vi "Combine Litho Data.vi"(8 "error in (no error)":errorcluster, 11 "Tool Object in":refnum<class "Tool Object.lvclass">) -> (0 "error out":errorcluster, 2 "Output":T1(array[cluster]), 3 "Tool Object out":refnum<class "Tool Object.lvclass">)   [LabVIEW 2019, in "Tool Object.lvclass"]
uses:
  Tool Object.lvclass
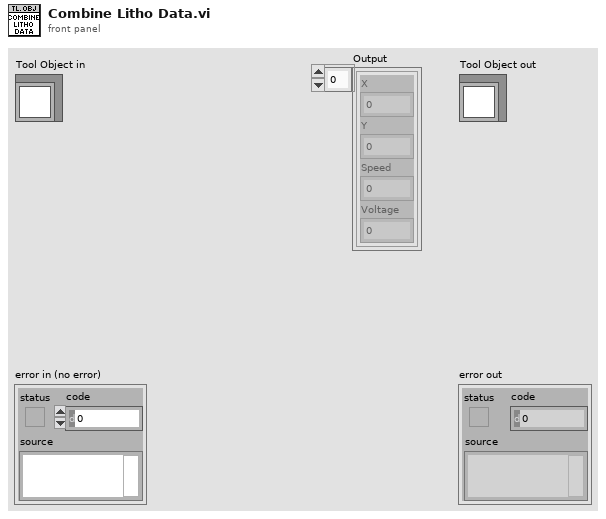
[diagram p1: front panel]
types:
  T1 = cluster{"X":dbl, "Y":dbl, "Speed":dbl, "Voltage":dbl}[]
  T2 = typedef "PathCommands.lvclass/Point.ctl" = cluster{"X":dbl, "Y":dbl}
  T3 = cluster{"X":dbl, "Y":dbl, "Speed":dbl, "Voltage":dbl}
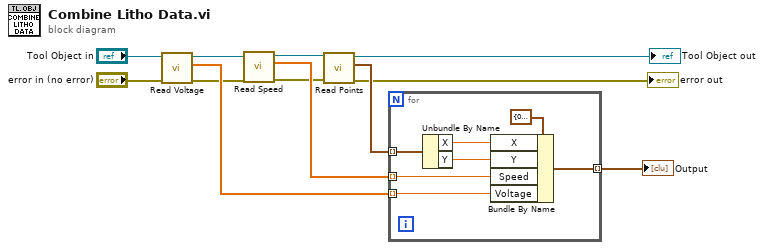
[diagram p0: block diagram]
diagram:
  n1 = call-dynamic "Read Voltage.vi"("error in (no error)"="error in (no error)", "Tool Object in"="Tool Object in") -> ("error out"=w4:errorcluster, "Voltage"=w6:dbl[], "Tool Object out"=w8:refnum<class "Tool Object.lvclass">)  [unwired: 7 in]
  n2 = call-dynamic "Read Speed.vi"("error in (no error)"=w4, "Tool Object in"=w8) -> ("error out"=w3:errorcluster, "Speed"=w5:dbl[], "Tool Object out"=w9:refnum<class "Tool Object.lvclass">)  [unwired: 7 in]
  n3 = call-dynamic "Read Points.vi"("error in (no error)"=w3, "Tool Object in"=w9) -> ("error out"=→"error out":errorcluster, "Points"=w12:T2[], "Tool Object out"=→"Tool Object out":refnum<class "Tool Object.lvclass">)  [unwired: 7 in]
  n4 = for {
    tunnel: w5 -> [w15] mode=indexing
    tunnel: w12 -> [w19] mode=indexing
    tunnel: w6 -> [w14] mode=indexing
    tunnel: [w13] -> w11 mode=indexing
    n5 = Unbundle By Name(w19) -> ("X"=w17:dbl, "Y"=w16:dbl)
    n6 = Bundle By Name(cluster=T3 {"X"=0.0, "Y"=0.0, "Speed"=0.0, "Voltage"=0.0} ("Litho Point"), "X"=w17, "Y"=w16, "Speed"=w15, "Voltage"=w14) -> (w13:T3)
  }
  "Output" <- w11
